vi "Divide XY (single).vi"(8 "error in (no error)":errorcluster, 10 "y":dbl, 11 "XY-data in":cluster{"X-array":dbl[], "Y-array":dbl[]}) -> (0 "error out":errorcluster, 3 "XY-data out":cluster{"X-array":dbl[], "Y-array":dbl[]} {"Y-array" format="%.2p"; "X-array" format="%.2p"})   [LabVIEW 2016, in "xy_utilities.lvlib"]
uses:
  xy_utilities.lvlib
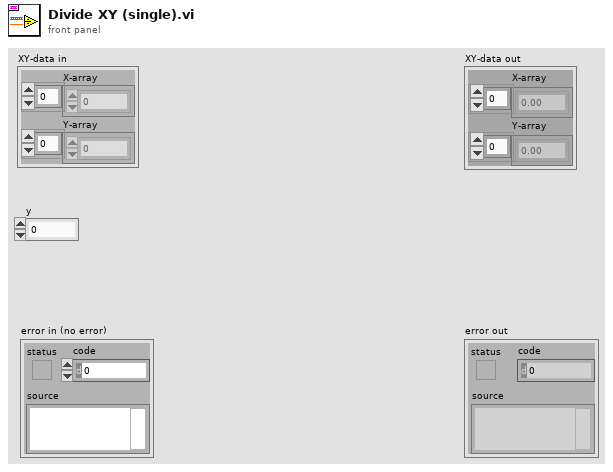
[diagram p1: front panel]
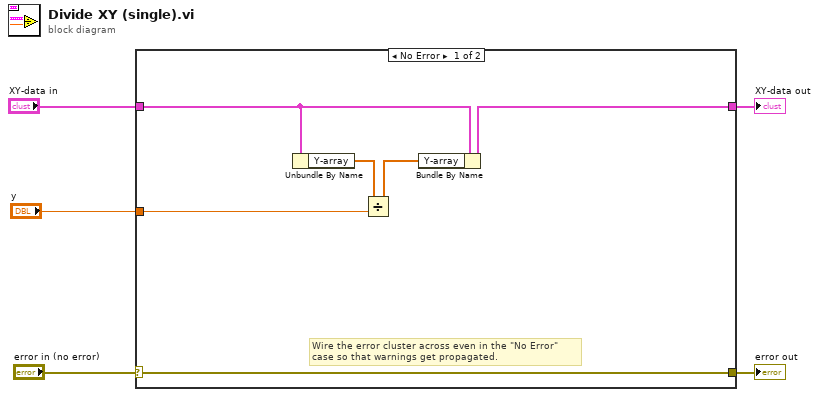
[diagram p0: block diagram]
diagram:
  n1 = case shown="No Error" "error in (no error)" {
    selector: "error in (no error)" -> [w11 w13]
    tunnel: [w11 w13] -> w4
    tunnel: "XY-data in" -> [w10 w12]
    tunnel: [w9 w12] -> w2
    tunnel: "y" -> [w7 _]
    frame No Error {
      # "Wire the error cluster across even in the \"No Error\"\ncase so that warnings get propagated."
      n2 = Unbundle By Name(w10) -> ("Y-array"=w8:dbl[])
      n3 = Divide(x=w8, y=w7) -> (x/y=w6:dbl[])
      n4 = Bundle By Name(cluster=w10, "Y-array"=w6) -> (w9:cluster{"X-array":dbl[], "Y-array":dbl[]})
    }
    frame Error {
    }
  }
  "error out" <- w4
  "XY-data out" <- w2
